vi "WriteMemory.vi"(8 "error in (no error)":errorcluster, 10 "Parameters":T1, 11 "Ref":T2) -> (0 "error out":errorcluster, 3 "Ref out":T2)   [LabVIEW 2024, in "Diagnostics Host Automation API.lvlib"]
uses:
  Diagnostics Host Automation API.lvlib
  Addon/Addon Shared/Types/HostAutomation.Ref.ctl
  <vilib>/NI/STM/TCP/TCP Connection Info.ctl
  <vilib>/NI/STM/SubVIs/MetaDataElement.ctl
  Addon/Addon Shared/Types/DTC.Codes.ctl
  Addon/Addon Shared/Types/Command.Memory.ctl
  <vilib>/NI/NI VeriStand Addon Network Comm/Shared/NI VeriStand Addon Network Comm Shared.lvlib
  Addon/Addon Shared/Diagnostics Addon Shared.lvlib
  <vilib>/NI/STM/NI STM.lvlib
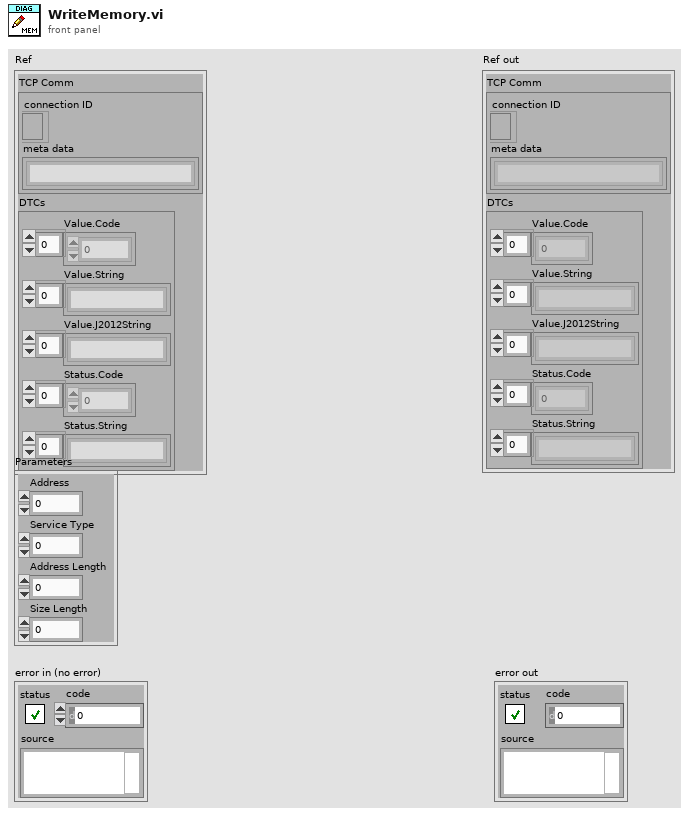
[diagram p1: front panel]
types:
  T1 = typedef "Diagnostics Addon Shared.lvlib/Command.Memory.ctl" = cluster{"Address":u64, "Service Type":u32, "Address Length":u8, "Size Length":u8}
  T2 = typedef "Diagnostics Addon Shared.lvlib/HostAutomation.Ref.ctl" = cluster{"TCP Comm":T3, "DTCs":T5}
  T3 = typedef "NI STM.lvlib/TCP Connection Info.ctl" = cluster{"connection ID":refnum<k5>, "meta data":T4[]}
  T4 = typedef "NI STM.lvlib/MetaDataElement.ctl" = string
  T5 = typedef "Diagnostics Addon Shared.lvlib/DTC.Codes.ctl" = cluster{"Value.Code":dbl[], "Value.String":string[], "Value.J2012String":string[], "Status.Code":dbl[], "Status.String":string[]}
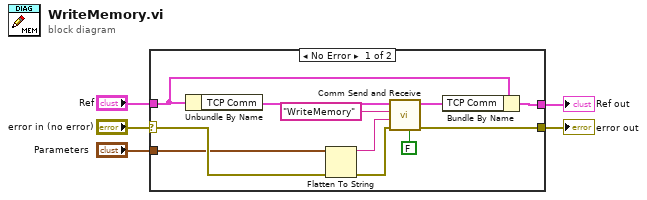
[diagram p0: block diagram]
diagram:
  n1 = case shown="No Error" "error in (no error)" {
    selector: "error in (no error)" -> [w13 w18]
    tunnel: "Ref" -> [w8 w17]
    tunnel: [w6 w17] -> w4
    tunnel: [w16 w18] -> w3
    tunnel: "Parameters" -> [w11 _]
    frame No Error {
      n2 = Unbundle By Name(w8) -> ("TCP Comm"=w9:T3)
      n3 = Flatten To String(anything=w11, error in (no error)=w13) -> (data string=w14:string, error out=w12:errorcluster)  [unwired: 2 in, 1 out]
      n4 = call <vilib>:"Comm Send and Receive.vi"("Resp Required?"=FALSE, "error in (no error)"=w12, "Data"=w14, "Name"="WriteMemory", "connection info"=w9) -> ("error out"=w16:errorcluster, "connection info"=w7:T3)  [unwired: 3 in, 2 out]
      n5 = Bundle By Name(cluster=w8, "TCP Comm"=w7) -> (w6:T2)
    }
    frame Error {
    }
  }
  "Ref out" <- w4
  "error out" <- w3
